vi "getFlow.vi"(2 "error in":errorcluster, 3 "AIN Range":u16(ring) items=["LJ_rgBIP10V", "LJ_rgBIP1V", "LJ_rgBIPP1V", "LJ_rgBIPP01V"], 4 "+ Channel":i32, 5 "Handle In":i32) -> (0 "error out":errorcluster, 1 "Voltage Reading":dbl format="%.6f")   [LabVIEW 2021]
panel:
  # "inputs"
  # "outputs"
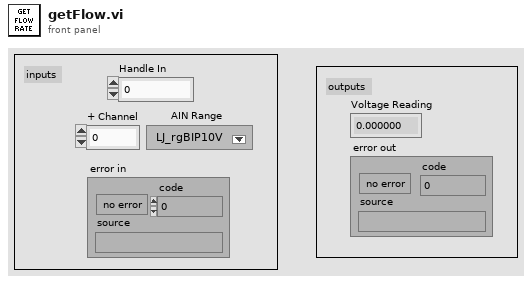
[diagram p1: front panel]
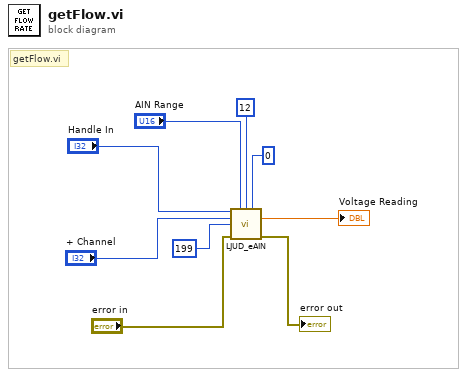
[diagram p0: block diagram]
diagram:
  # "getFlow.vi"
  n1 = call <vilib>:"LJUD_eAIN.vi"("Handle In"="Handle In", "Range"="AIN Range", "Resolution"=12, "Settling"=0, "ChannelP"="+ Channel", "ChannelN"=199, "error in"="error in") -> ("Voltage"=→"Voltage Reading":dbl, "error out"=→"error out":errorcluster)  [unwired: 6 in, 1 out]
